vi "Query PORT output modes.vi"(8 "error in (no error)":errorcluster, 10 "i (0)":T2, 11 "VISA resource name":refnum<visa-resource-name>) -> (0 "error out":errorcluster, 2 "output":T1, 3 "VISA resource name out":refnum<visa-resource-name>)   [LabVIEW 2009, in "SR400.lvlib"]
doc: "PM i { ,j }\nThe PM command sets and reads the rear panel\nPORT1 and PORT2 D/A output modes. i=1 or 2\nto select PORT1 or PORT 2 and is required. If j is\nincluded, the mode is set to FIXED, j=0, or\nSCAN, j=1. If j is absent, the mode is returned.\nThe mode may be changed during a scan. If it is\nchanged to SCAN, the level begins scanning from\nthe start value on the next count period. If it is\nchanged to FIXED, the level returns to the start\nvalue immediately."
uses:
  SR400.lvlib
  Typedefs.llb/PORT Output.ctl
  Typedefs.llb/Discriminator Output.ctl
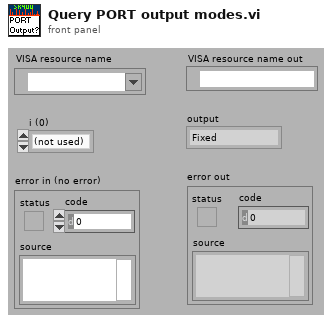
[diagram p1: front panel]
types:
  T1 = typedef "SR400.lvlib/Discriminator Output.ctl" = enum16{"Fixed", "Scan"}
  T2 = typedef "SR400.lvlib/PORT Output.ctl" = enum16{"(not used)", "PORT 1", "PORT 2"}
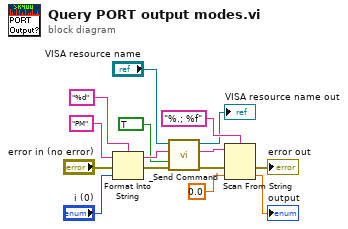
[diagram p0: block diagram]
diagram:
  n1 = Format Into String(format string="%d", initial string="PM" ("command"), error in="error in (no error)", "i (0)") -> (resulting string=w6:string, error out=w5:errorcluster)
  n2 = call "_Send Command.vi"("error in (no error)"=w5, "Query? (F)"=TRUE, "Command"=w6, "VISA resource name"="VISA resource name") -> ("error out"=w2:errorcluster, "Response"=w3:string, "VISA resource name out"=→"VISA resource name out":refnum<visa-resource-name>)  [unwired: 5 out]
  n3 = Scan From String(format string="%.; %f", input string=w3, error in=w2, default 1=0.0 ("default value 1")) -> (error out=→"error out":errorcluster, output 1=→"output":dbl)  [unwired: 1 in, 2 out]
